vi "设置字体.vi"(8 "error in (no error)":errorcluster caption="错误输入（无错误）", 11 "程序 输入":refnum<class "程序.lvclass">) -> (0 "error out":errorcluster caption="错误输出", 3 "程序 输出":refnum<class "程序.lvclass">)   [LabVIEW 2020, in "程序.lvclass"]
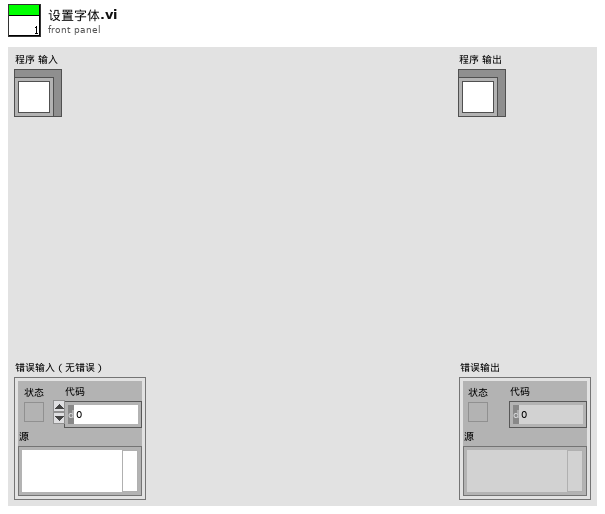
[diagram p1: front panel]
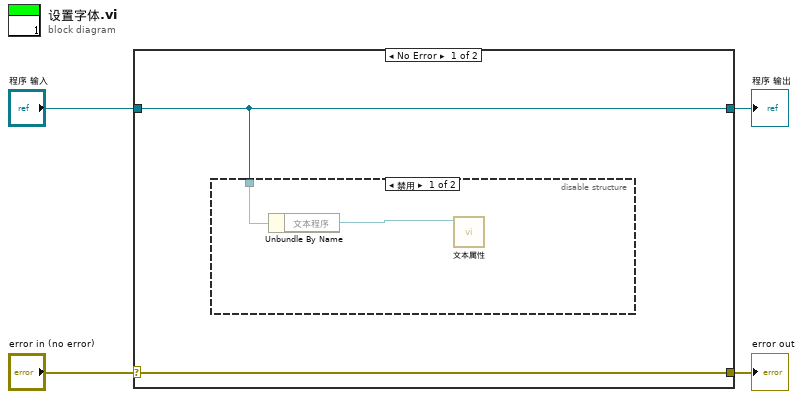
[diagram p0: block diagram]
diagram:
  n1 = case shown="No Error" "error in (no error)" {
    selector: "error in (no error)" -> [w6 w10]
    tunnel: [w6 w10] -> w3
    tunnel: [w5 w9] -> w1
    tunnel: "程序 输入" -> [w5 w9]
    frame No Error {
      n2 = disable-structure shown="禁用" {
        disable-tunnel: w5 -> [w8 _]
        frame Disabled {
          n3 = Unbundle By Name(w8) -> ("文本程序"=w7:refnum<vi>)
          n4 = call "文本属性.vi"("引用"=w7) -> ()  [unwired: 11 in]
        }
        frame Enabled {
        }
      }
    }
    frame Error {
    }
  }
  "error out" <- w3
  "程序 输出" <- w1
